vi "clear_buffers.vi"(8 "error in (no error)":errorcluster, 11 "FPGAWrapperRK110909Throughput in":refnum<class "FPGAWrapperRK110909Throughput.lvclass">) -> (0 "error out":errorcluster, 3 "FPGAWrapperRK110909Throughput out":refnum<class "FPGAWrapperRK110909Throughput.lvclass">)   [LabVIEW 2010, in "FPGAWrapperRK110909Throughput.lvclass"]
uses:
  FPGAWrapperRK110909Throughput.lvclass
  <vilib>/rvi/interface/nirviMethod/nirviMethod.xnode
  FPGA_reference.ctl
  <vilib>/Utility/error.llb/Error Cluster From Error Code.vi
  NiFpgaLv.dll
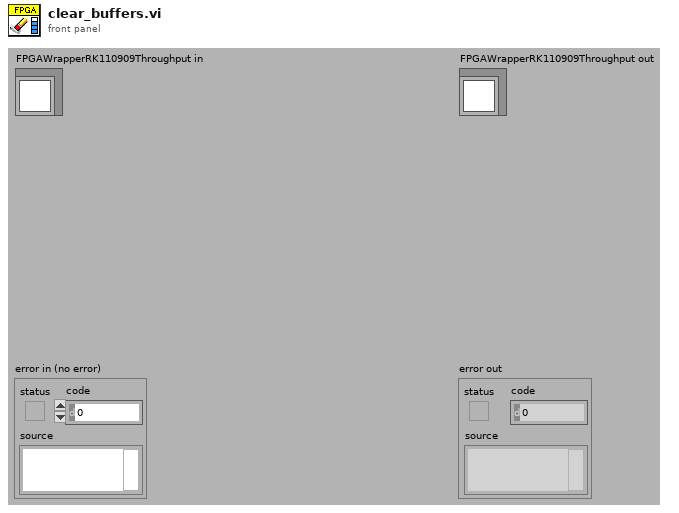
[diagram p1: front panel]
types:
  T1 = typedef "FPGAWrapperRK110909Throughput.lvclass/FPGA_reference.ctl" = refnum<k20>
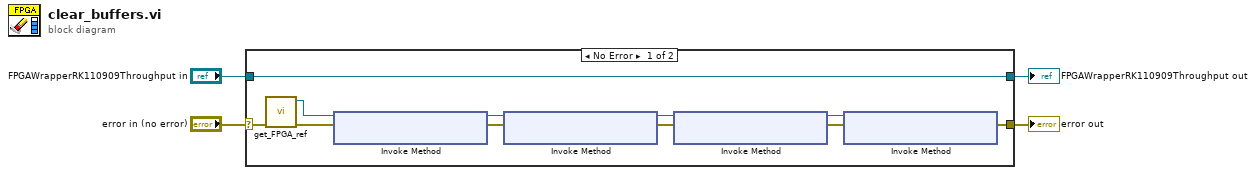
[diagram p0: block diagram]
diagram:
  n1 = case shown="No Error" "error in (no error)" {
    selector: "error in (no error)" -> [w6 w104]
    tunnel: [w7 w104] -> w4
    tunnel: "FPGAWrapperRK110909Throughput in" -> [w5 w105]
    tunnel: [w5 w105] -> w1
    frame No Error {
      n2 = call "get_FPGA_ref.vi"("error in"=w6) -> ("error out"=w9:errorcluster, "FPGA Reference"=w8:T1)  [unwired: 8 in, 1 out]
      n3 = xnode "Invoke Method"("FPGA VI Reference In"=w8, "error in"=w9) -> ("FPGA VI Reference Out"=w14:T1, "error out"=w15:errorcluster)
      n4 = xnode "Invoke Method"("FPGA VI Reference In"=w14, "error in"=w15) -> ("FPGA VI Reference Out"=w12:T1, "error out"=w13:errorcluster)
      n5 = xnode "Invoke Method"("FPGA VI Reference In"=w12, "error in"=w13) -> ("FPGA VI Reference Out"=w10:T1, "error out"=w11:errorcluster)
      n6 = xnode "Invoke Method"("FPGA VI Reference In"=w10, "error in"=w11) -> ("error out"=w7:errorcluster)  [unwired: 1 out]
    }
    frame Error {
    }
  }
  "error out" <- w4
  "FPGAWrapperRK110909Throughput out" <- w1
